vi "(FPGA)_PIDXYZ_laserPID)_COMtemp2.vi"() -> ()   [LabVIEW 2018]
doc: "This VI will read single point values from 4 channels of a R Series board at a specified rate."
uses:
  <vilib>/rvi/Emulation/niFpgaGetClockAttributes.vi
  <vilib>/rvi/Emulation/niFpgaSctlEmulationGetInTimedLoop.vi
  <vilib>/rvi/Emulation/niFpgaEmulationReportErrorSimple.vi
  <vilib>/rvi/eio/common/nirviEmuTemplateMethod_errors.vi
  <vilib>/rvi/Emulation/niFpgaProcessEmulError.vi
  <vilib>/rvi/Emulation/niFpgaCriticalErrorInLSC.vi
  <vilib>/rvi/Memory/Memory_Emulation/nirvimemoryFastEmulation.vi
  <vilib>/rvi/Memory/Memory_Emulation/nirvimemoryEmulation.vi
  <vilib>/rvi/Emulation/niFpgaEmulationIsFPGAContextNoSignature.vi
  <vilib>/rvi/DataTransferAndStorage/Container/Common/niFpgaContainerGetUniqueNameForEmu.vi
  <vilib>/rvi/errors/nirviReportUnexpectedCaseInternalError (U32).vi
  <vilib>/rvi/Memory/Memory_Emulation/niFpgaMemoryEmulationCacheClearOnFirstRun.vi
  <vilib>/rvi/Memory/Memory_Emulation/nirvimemoryEmulationManagerCache_MakeExclusive.vi
  <vilib>/rvi/Memory/Memory_Emulation/niFpgaMemoryEmulationValidateCache.vi
  <vilib>/rvi/Memory/Memory_Emulation/nirvimemoryEmulationManagerCache_InsertValue.vi
  <vilib>/Utility/error.llb/Clear Errors.vi
  <vilib>/rvi/Memory/Memory_Emulation/nirvimemoryEmulationManagerCache_ReleaseExclusive.vi
  <vilib>/rvi/Memory/Memory_Emulation/nirvimemoryEmulationManagerCache_GetValue.vi
  <vilib>/rvi/Memory/Memory_Emulation/nirvimemoryEmulationManagerCache_SetValue.vi
  <vilib>/rvi/Emulation/niFpgaSctlEmulationResourceMgr.vi
  <vilib>/eio/EIONode/EIONode.xnode
  <vilib>/rvi/DataTransferAndStorage/Container/XNode/niFpgaContainer.xnode
  <vilib>/rvi/FXPMathLib/FxpInterpret/XNode/nifxpmath_Interpret.xnode
panel:
  in  "Amplitude AO7":fxp<+/-,64,32>
  in  "Amplitude AO6":fxp<+/-,64,32>
  in  "Amplitude AO5":fxp<+/-,64,32>
  in  "Amplitude AO4":fxp<+/-,64,32>
  in  "phase offset AO7":fxp<+,32,0>
  in  "reset AO7":bool
  in  "frequency AO7":fxp<+,32,0>=0.0002500000409781933
  in  "phase offset AO6":fxp<+,32,0>
  in  "reset AO6":bool
  in  "frequency AO6":fxp<+,32,0>=0.0002500000409781933
  in  "phase offset AO5":fxp<+,32,0>
  in  "reset AO5":bool
  in  "frequency AO5":fxp<+,32,0>=0.0002500000409781933
  in  "phase offset AO4":fxp<+,32,0>
  in  "reset AO4":bool
  in  "frequency AO4":fxp<+,32,0>=0.0002500000409781933
  in  "stop":bool
  in  "Notch coeff y 2":i32[](array[numeric])=[-1060332860, 1067037342, -2129863576]
  in  "Notch coeff y 1":i32[](array[numeric])=[-1060332860, 1067037342, -2129863576]
  in  "Notch coeff x":i32[](array[numeric])=[-1060332860, 1067037342, -2129863576]
  out "accum out z2":fxp<+/-,37,37>
  out "accurm reset z2":bool
  out "accum out z1":fxp<+/-,37,37>
  out "accum reset z1":bool
  in  "Reset x accum":bool
  in  "Reset y accum":bool
  in  "Reset z accum":bool
  out "master y":bool
  out "master x":bool
  in  "No_integral_gain":bool=TRUE
  in  "Y_emergency_threshould":i16
  in  "X_emergency_threshould":i16
  in  "Big Number":sgl
  in  "Amplitude_sine_EOM":sgl
  in  "eom sine frequency (periods/tick)":fxp<+,32,0>=0.0002500000409781933
  in  "pz?":bool
  out "pg Z mod":fxp<+/-,24,12>
  in  "pg Z":fxp<+/-,24,12>
  in  "amplitude":i16=8192
  in  "offset":i16=8192
  out "Trigger for COM out":i16 caption="square wave out"
  out "dgz mod":fxp<+/-,24,12>
  in  "activate COMz":bool
  in  "dg Z":fxp<+/-,24,12>
  in  "activate COMy":bool
  out "dgy mod":fxp<+/-,24,12>
  in  "dg Y":fxp<+/-,24,12>
  out "dgx mod":fxp<+/-,24,12>
  in  "activate COMx":bool
  in  "dg X":fxp<+/-,24,12>
  in  "duty cycle (periods)":fxp<+,32,0>=0.5
  in  "frequency (periods/tick)":fxp<+,32,0>=0.00390625
  in  "final filter coeff X before":i32[](array[numeric])=[-955995012, 2025731616, 1001305, -1023351008, 2092954700, 1034533]
  in  "final filter coeff X":i32[](array[numeric])=[-955995012, 2025731616, 1001305, -1023351008, 2092954700, 1034533]
  in  "final filter coeff Y before":i32[](array[numeric])=[-955995012, 2025731616, 1001305, -1023351008, 2092954700, 1034533]
  in  "final filter coeff Y":i32[](array[numeric])=[-955995012, 2025731616, 1001305, -1023351008, 2092954700, 1034533]
  in  "final filter coeff Z":i32[](array[numeric])=[-955995012, 2025731616, 1001305, -1023351008, 2092954700, 1034533]
  in  "final filter coeff Z before":i32[](array[numeric])=[-955995012, 2025731616, 1001305, -1023351008, 2092954700, 1034533]
  in  "LP Coeff Z before":i32[](array[numeric])=[1008310688, 32715568]
  in  "LP Coeff Z":i32[](array[numeric])=[1008310688, 32715568]
  in  "LP Coeff X":i32[](array[numeric])=[1008310688, 32715568]
  in  "LP Coeff X before":i32[](array[numeric])=[1008310688, 32715568]
  in  "LP Coeff Y before":i32[](array[numeric])=[1008310688, 32715568]
  in  "LP Coeff Y":i32[](array[numeric])=[1008310688, 32715568]
  in  "Upper lim Z before":fxp<+/-,16,16>
  in  "Lower lim Z before":fxp<+/-,16,16>
  in  "Upper lim Y before":fxp<+/-,16,16>
  in  "Lower lim Y before":fxp<+/-,16,16>
  in  "Upper lim X before":fxp<+/-,16,16>
  in  "Lower lim X before":fxp<+/-,16,16>
  in  "HP coeff band X before":i32[](array[numeric])=[-850883994, 1909449570, 958518847, -975456236, 2033039520, 1020559395]
  in  "LP Coeff band X before":i32[](array[numeric])=[-955995012, 2025731616, 1001305, -1023351008, 2092954700, 1034533]
  in  "LP Coeff band X":i32[](array[numeric])=[-955995012, 2025731616, 1001305, -1023351008, 2092954700, 1034533]
  in  "HP Coeff band X":i32[](array[numeric])=[-850883994, 1909449570, 958518847, -975456236, 2033039520, 1020559395]
  in  "dg band X before":fxp<+/-,24,12>
  in  "dg band X":fxp<+/-,24,12>
  in  "HP Coeff X before":i32[](array[numeric])=[946630756, 1010186290]
  in  "HP Coeff X":i32[](array[numeric])=[946630756, 1010186290]
  in  "Use X PID before":bool
  out "AI X before chamber plot":i16
  in  "X before Setpoint":i16
  out "tot_fb X plot":i16
  out "fb X before chamber plot":i16
  in  "DC offset X":i16
  in  "pg X before":fxp<+/-,24,12>
  in  "ig X before":fxp<+/-,24,-4>
  in  "dg X before":fxp<+/-,24,12>
  out "fb X plot":i16
  in  "ig X":fxp<+/-,24,-4>
  in  "Lower lim X":fxp<+/-,16,16>
  in  "Upper lim X":fxp<+/-,16,16>
  in  "pg X":fxp<+/-,24,12>
  out "AI X plot":i16
  in  "X Setpoint":i16
  in  "HP coeff band Y before":i32[](array[numeric])=[-850883994, 1909449570, 958518847, -975456236, 2033039520, 1020559395]
  in  "LP Coeff band Y before":i32[](array[numeric])=[-955995012, 2025731616, 1001305, -1023351008, 2092954700, 1034533]
  in  "LP Coeff band Y":i32[](array[numeric])=[-955995012, 2025731616, 1001305, -1023351008, 2092954700, 1034533]
  in  "HP Coeff band Y":i32[](array[numeric])=[-850883994, 1909449570, 958518847, -975456236, 2033039520, 1020559395]
  in  "dg band Y before":fxp<+/-,24,12>
  in  "dg band Y":fxp<+/-,24,12>
  in  "HP Coeff Y before":i32[](array[numeric])=[946630756, 1010186290]
  in  "HP Coeff Y":i32[](array[numeric])=[946630756, 1010186290]
  in  "Use Y PID before":bool
  out "AI Y before chamber plot":i16
  in  "Y before Setpoint":i16
  out "tot_fb Y plot":i16
  out "fb Y before chamber plot":i16
  in  "DC offset Y":i16
  in  "pg Y before":fxp<+/-,24,12>
  in  "ig Y before":fxp<+/-,24,-4>
  in  "dg Y before":fxp<+/-,24,12>
  out "fb Y plot":i16
  in  "ig Y":fxp<+/-,24,-4>
  in  "Lower lim Y":fxp<+/-,16,16>
  in  "Upper lim Y":fxp<+/-,16,16>
  in  "pg Y":fxp<+/-,24,12>
  out "AI Y plot":i16
  in  "Y Setpoint":i16
  in  "EOM_offset":i16
  in  "EOM_seed":u32=4294967295 caption="seed"
  in  "EOM reset":bool caption="reset"
  in  "EOM_threshold":i16
  in  "EOM_amplitude":i16
  in  "HP coeff band Z before":i32[](array[numeric])=[-850883994, 1909449570, 958518847, -975456236, 2033039520, 1020559395]
  in  "LP Coeff band Z before":i32[](array[numeric])=[-955995012, 2025731616, 1001305, -1023351008, 2092954700, 1034533]
  in  "LP Coeff band Z":i32[](array[numeric])=[-955995012, 2025731616, 1001305, -1023351008, 2092954700, 1034533]
  in  "HP Coeff band Z":i32[](array[numeric])=[-850883994, 1909449570, 958518847, -975456236, 2033039520, 1020559395]
  in  "dg band Z before":fxp<+/-,24,12>
  in  "dg band Z":fxp<+/-,24,12>
  in  "data_buffer3":i16
  in  "Arb gain (ch2)":fxp<+/-,24,12>=0.5 caption="RMS"
  in  "HP Coeff Z before":i32[](array[numeric])=[946630756, 1010186290]
  in  "HP Coeff Z":i32[](array[numeric])=[946630756, 1010186290]
  in  "Use Z PID before":bool
  out "AI Z before chamber plot":i16
  in  "Z before Setpoint":i16
  out "tot_fb Z plot":i16
  out "fb Z before chamber plot":i16
  in  "DC offset Z":i16
  in  "pg Z before":fxp<+/-,24,12>
  in  "ig Z before":fxp<+/-,24,-4>
  in  "dg Z before":fxp<+/-,24,12>
  out "fb Z plot":i16
  in  "ig Z":fxp<+/-,24,-4>
  out "written_address":u32
  in  "ready_to_write":bool
  in  "Arb steps per cycle":u16
  in  "data_buffer2":i16
  in  "data_buffer_1":i16
  in  "write_address":u16
  in  "Arb gain (ch1)":fxp<+/-,24,12>=0.5 caption="RMS"
  in  "Arb gain (ch0)":fxp<+/-,24,12>=0.5 caption="RMS"
  in  "Lower lim Z":fxp<+/-,16,16>
  in  "Upper lim Z":fxp<+/-,16,16>
  out "AI Z plot":i16
  in  "Z Setpoint":i16
  in  "Count(uSec)":u32
  out "FPGA Error Out":errorcluster
  in  "Stop":bool
  # "test"
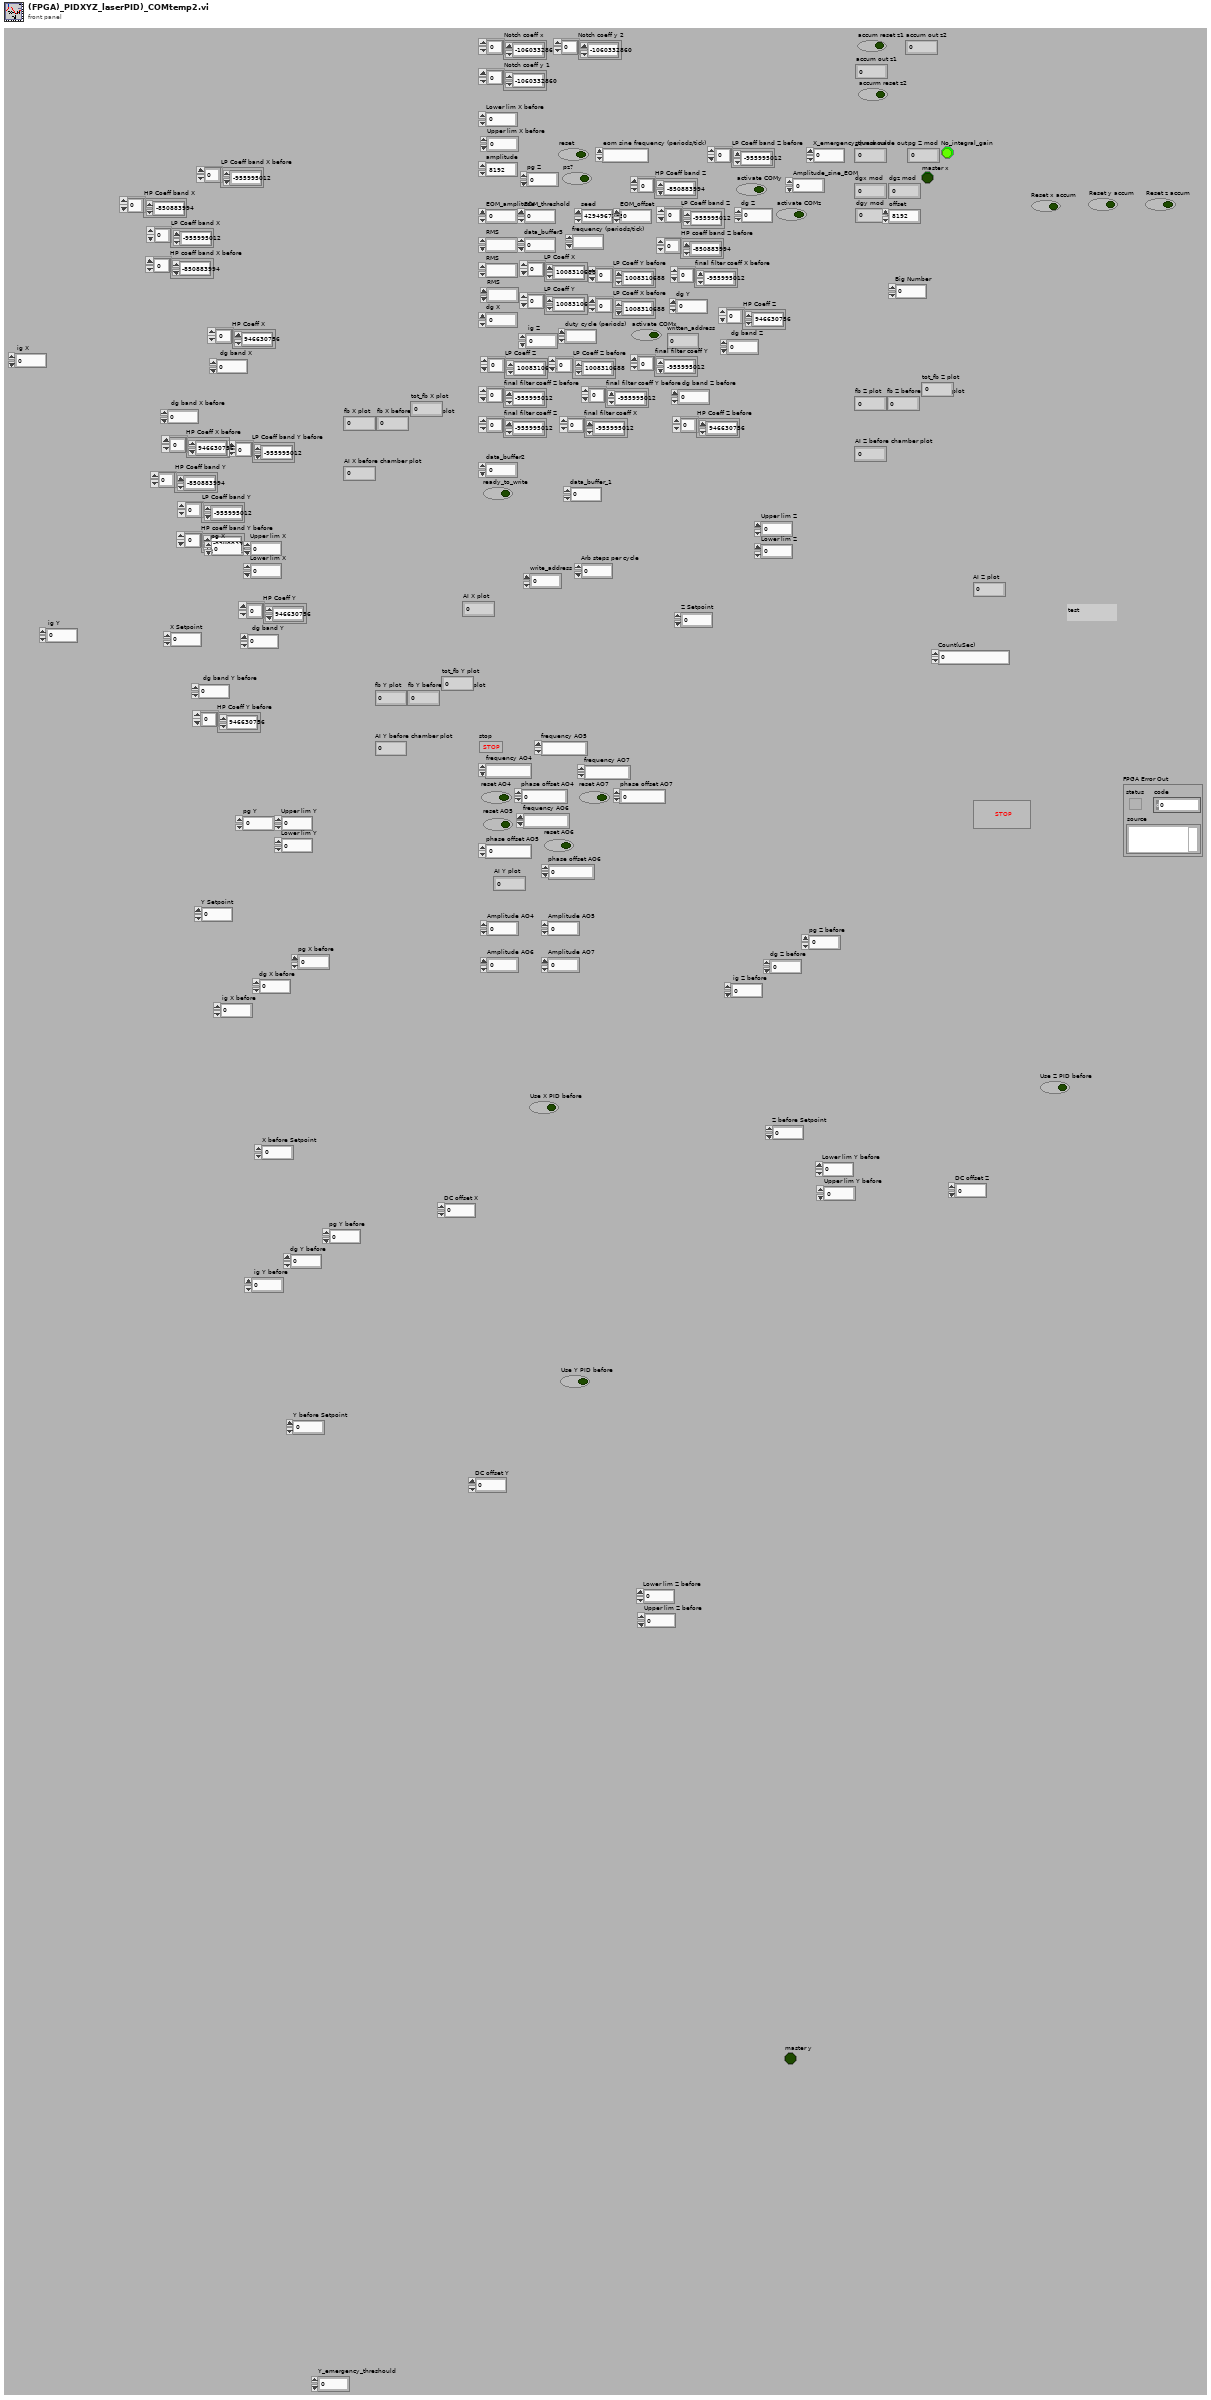
[diagram p1: front panel]
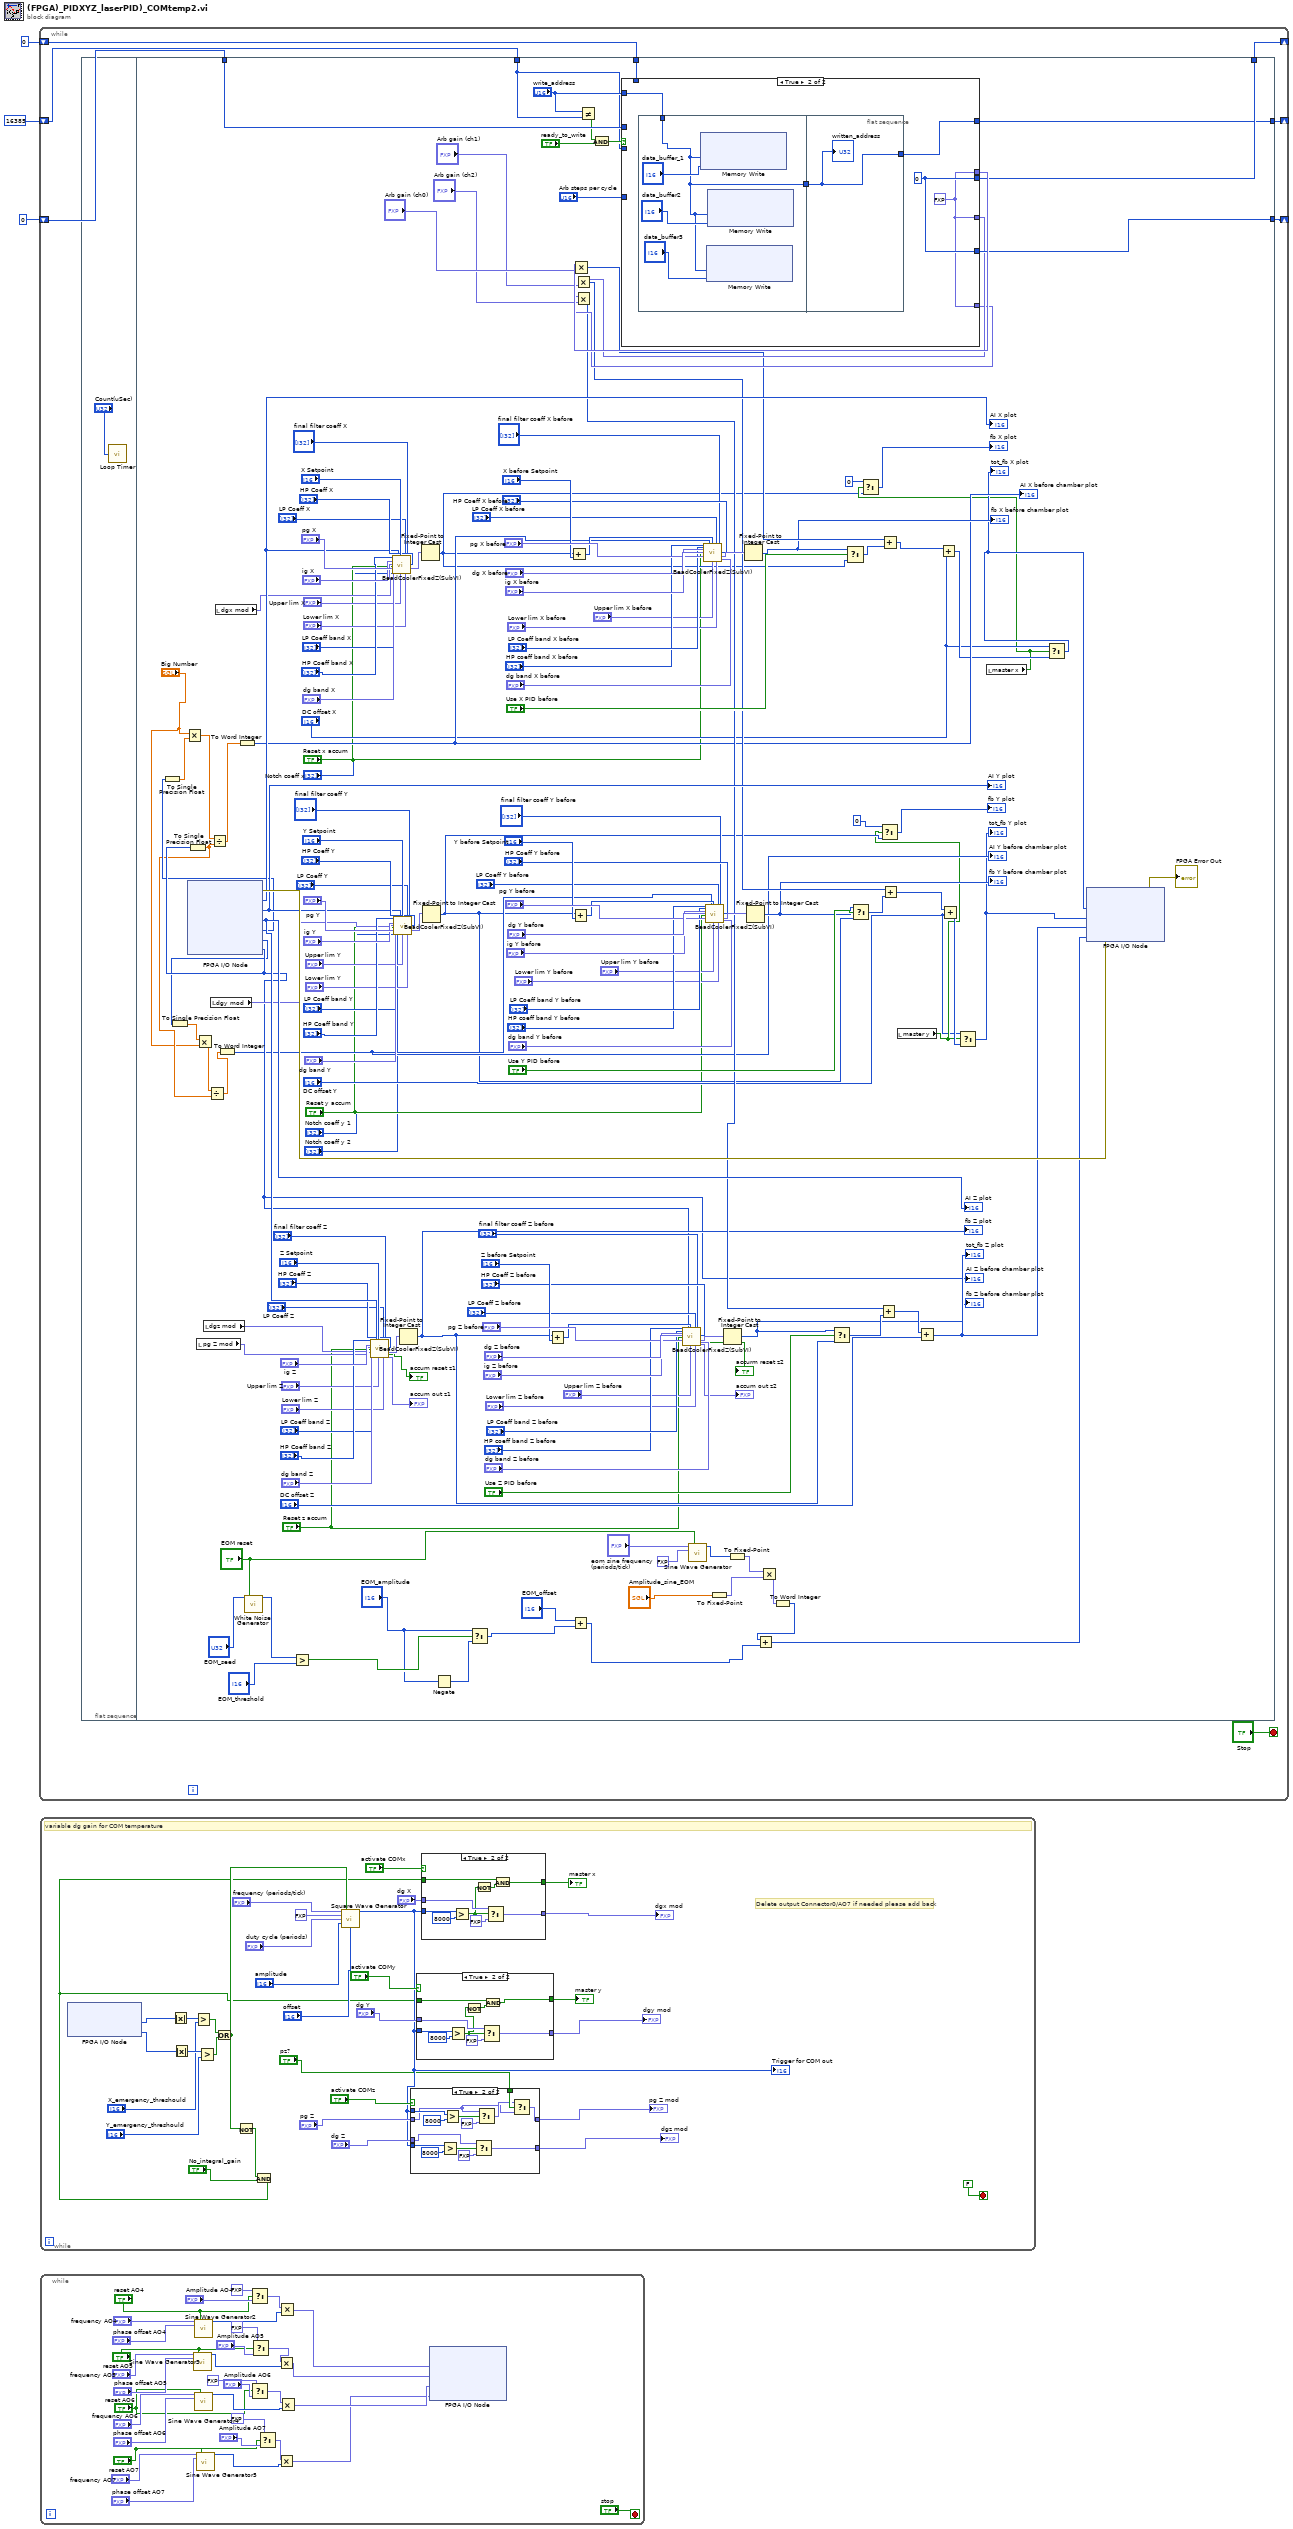
[diagram p0: block diagram]
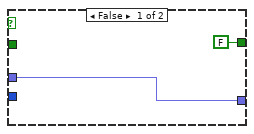
[diagram p3: hidden frame]
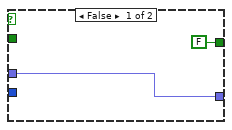
[diagram p4: hidden frame]
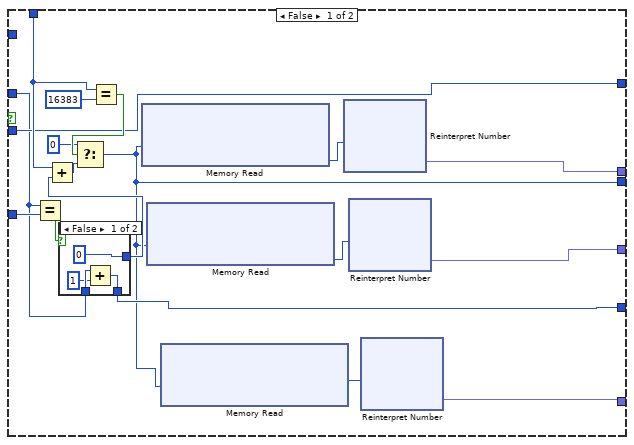
[diagram p5: hidden frame]
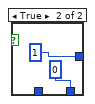
[diagram p6: hidden frame]
diagram:
  n1 = while {
    shift-right: [w9] -> _
    shift-left: u16 0 ("t") -> [w8]
    shift-right: [w7] -> _
    shift-left: u16 0 ("t") -> [w4]
    shift-right: [w6] -> _
    shift-left: u32 16385 ("write_address") -> [w5]
    stop <- "Stop" stop-if-true
    n2 = flat-sequence {
      tunnel: [w183] -> w9
      tunnel: w8 -> [w182]
      tunnel: [w180] -> w7
      tunnel: w4 -> [w179]
      tunnel: [w178] -> w6
      tunnel: w5 -> [w171]
      frame #0 {
        n3 = call "Loop Timer"("Count(uSec)"="Count(uSec)") -> ()  [unwired: 1 out]
      }
      frame #1 {
        n4 = xnode "FPGA I/O Node"() -> ("error out"=w188:errorcluster, "Connector0/AI0"=w95:i16, "Connector0/AI1"=w117:i16, "Connector0/AI2"=w169:i16, "Connector0/AI3"=w43:i16, "Connector0/AI4"=w42:i16, "Connector0/AI5"=w47:i16)  [unwired: 7 in, 6 out]
        "AI Z plot" <- w169
        "AI Z before chamber plot" <- w47
        "AI Y plot" <- w117
        "AI X plot" <- w95
        n5 = To Single Precision Float(number=w43) -> (single precision float=w46:sgl)
        n6 = To Single Precision Float(number=w42) -> (single precision float=w41:sgl)
        n7 = Multiply(x="Big Number", y=w46) -> (x*y=w45:sgl)
        n8 = To Single Precision Float(number=w47) -> (single precision float=w39:sgl)
        n9 = Multiply(x=w41, y="Big Number") -> (x*y=w40:sgl)
        n10 = local read "pg Z mod"() -> (w60:fxp<+/-,24,12>)
        n11 = local read "dgz mod"() -> (w61:fxp<+/-,24,12>)
        n12 = Divide(x=w40, y=w39) -> (x/y=w38:sgl)
        n13 = Divide(x=w45, y=w39) -> (x/y=w44:sgl)
        n14 = local read "dgy mod"() -> (w62:fxp<+/-,24,12>)
        n15 = local read "dgx mod"() -> (w63:fxp<+/-,24,12>)
        n16 = To Word Integer(number=w38) -> (16bit integer=w37:i16)
        "AI Y before chamber plot" <- w37
        n17 = To Word Integer(number=w44) -> (16bit integer=w48:i16)
        "AI X before chamber plot" <- w48
        n18 = call "White Noise Generator"("seed"="EOM_seed", "reset"="EOM reset") -> ("white noise out"=w148:i16)  [unwired: 13 in]
        n19 = Greater?(x=w148, y="EOM_threshold") -> (0:w146:bool)
        n20 = call "BeadCoolerFixedZ(SubVI).vi"("hp coeff band"="HP Coeff band Z", "lp coeff band"="LP Coeff band Z", "ig"="ig Z", "dg"=w61, "load (F)"="Reset z accum", "pg"=w60, "dg band"="dg band Z", "AI0"=w169, "Dc Pos"="Z Setpoint", "Upper lim"="Upper lim Z", "lp coeff"="LP Coeff Z", "Lower lim"="Lower lim Z", "final filter coeff"="final filter coeff Z", "hp coeff"="HP Coeff Z") -> ("Output"=w158:fxp<+/-,16,16>, "accurm reset"=→"accum reset z1":bool, "accum out"=→"accum out z1":fxp<+/-,37,37>)  [unwired: 11 in]
        n21 = call "BeadCoolerFixedZ(SubVI).vi"("hp coeff band"="HP Coeff band X", "lp coeff band"="LP Coeff band X", "ig"="ig X", "dg"=w63, "load (F)"="Reset x accum", "pg"="pg X", "dg band"="dg band X", "Notch coeff 1"="Notch coeff x", "AI0"=w95, "Dc Pos"="X Setpoint", "Upper lim"="Upper lim X", "lp coeff"="LP Coeff X", "Lower lim"="Lower lim X", "final filter coeff"="final filter coeff X", "hp coeff"="HP Coeff X") -> ("Output"=w105:fxp<+/-,16,16>)  [unwired: 10 in, 2 out]
        n22 = call "BeadCoolerFixedZ(SubVI).vi"("hp coeff band"="HP Coeff band Y", "lp coeff band"="LP Coeff band Y", "ig"="ig Y", "dg"=w62, "load (F)"="Reset y accum", "pg"="pg Y", "dg band"="dg band Y", "Notch coeff 1"="Notch coeff y 1", "Notch coeff 2"="Notch coeff y 2", "AI0"=w117, "Dc Pos"="Y Setpoint", "Upper lim"="Upper lim Y", "lp coeff"="LP Coeff Y", "Lower lim"="Lower lim Y", "final filter coeff"="final filter coeff Y", "hp coeff"="HP Coeff Y") -> ("Output"=w127:fxp<+/-,16,16>)  [unwired: 9 in, 2 out]
        n23 = Fixed-Point to Integer Cast(1:w158) -> (0:w73:i16)
        "fb Z plot" <- w73
        n24 = Fixed-Point to Integer Cast(1:w105) -> (0:w23:i16)
        n25 = Fixed-Point to Integer Cast(1:w127) -> (0:w31:i16)
        n26 = Negate(x="EOM_amplitude") -> (-x=w144:i16)
        n27 = Select(t="EOM_amplitude", s=w146, f=w144) -> (s? t:f=w142:i16)
        n28 = Add(x=w73, y="Z before Setpoint") -> (x+y=w157:i16)
        n29 = Add(x=w23, y="X before Setpoint") -> (x+y=w104:i16)
        n30 = Add(x=w31, y="Y before Setpoint") -> (x+y=w126:i16)
        n31 = Add(x="EOM_offset", y=w142) -> (x+y=w51:i16)
        n32 = Not Equal?(x="write_address", y=w171) -> (x != y?=w175:bool)
        n33 = And(x=w175, y="ready_to_write") -> (x .and. y?=w176:bool)
        n34 = case shown="True" w176 {
          tunnel: [w205 w213] -> w185
          tunnel: [w190 w217] -> w183
          tunnel: w182 -> [w198 _]
          tunnel: [w199 w213] -> w173
          tunnel: "Arb steps per cycle" -> [w197 _]
          tunnel: [w192 w217] -> w180
          tunnel: w179 -> [w193 _]
          tunnel: [w196 w215] -> w178
          tunnel: w171 -> [w196 _]
          tunnel: "write_address" -> [_ w214]
          tunnel: [w189 w213] -> w155
          frame False {
            n35 = Equal?(x=w193, y=w197) -> (x = y?=w195:bool)
            n36 = case shown="False" w195 {
              tunnel: [u16 0 ("y") u16 1 ("y")] -> w194
              tunnel: w193 -> [w209 _]
              tunnel: [w207 u16 0] -> w192
              frame False {
                n37 = Add(x=w209, y=u16 1) -> (x+y=w207:u16)
              }
              frame True {
              }
            }
            n38 = Add(x=w198, y=w194) -> (x+y=w201:u16)
            n39 = Equal?(x=w198, y=u16 16383) -> (x = y?=w203:bool)
            n40 = Select(t=u16 0, s=w203, f=w201) -> (s? t:f=w190:u16)
            n41 = xnode ("Memory Read")("Address"=w190) -> ("Data"=w206:i16)  [unwired: 1 in, 1 out]
            n42 = xnode ("Memory Read")("Address"=w190) -> ("Data"=w200:i16)  [unwired: 1 in, 1 out]
            n43 = xnode ("Memory Read")("Address"=w190) -> ("Data"=w191:i16)  [unwired: 1 in, 1 out]
            n44 = xnode "Reinterpret Number"("x"=w206) -> ("y"=w205:fxp<+/-,16,16>)
            n45 = xnode "Reinterpret Number"("x"=w200) -> ("y"=w199:fxp<+/-,16,16>)
            n46 = xnode "Reinterpret Number"("x"=w191) -> ("y"=w189:fxp<+/-,16,16>)
          }
          frame True {
            w217 = u16 0
            w213 = fxp<+/-,16,16> 0.0 ("y")
            n47 = flat-sequence {
              tunnel: [w219] -> w216
              tunnel: w214 -> [w219]
              tunnel: w216 -> [w222]
              tunnel: [w222] -> w215
              frame #0 {
                n48 = xnode ("Memory Write")("Address"=w219, "Data"="data_buffer_1") -> ()  [unwired: 1 in, 1 out]
                n49 = xnode ("Memory Write")("Address"=w219, "Data"="data_buffer3") -> ()  [unwired: 1 in, 1 out]
                n50 = xnode ("Memory Write")("Address"=w219, "Data"="data_buffer2") -> ()  [unwired: 1 in, 1 out]
              }
              frame #1 {
                "written_address" <- w222
              }
            }
          }
        }
        n51 = Multiply(x=w185, y="Arb gain (ch0)") -> (x*y=w76:i16)
        n52 = Multiply(x=w173, y="Arb gain (ch1)") -> (x*y=w75:i16)
        n53 = Multiply(x=w155, y="Arb gain (ch2)") -> (x*y=w74:i16)
        n54 = call "BeadCoolerFixedZ(SubVI).vi"("hp coeff band"="HP coeff band Z before", "lp coeff band"="LP Coeff band Z before", "ig"="ig Z before", "dg"="dg Z before", "load (F)"="Reset z accum", "pg"="pg Z before", "dg band"="dg band Z before", "AI0"=w47, "Dc Pos"=w157, "Upper lim"="Upper lim Z before", "lp coeff"="LP Coeff Z before", "Lower lim"="Lower lim Z before", "final filter coeff"="final filter coeff Z before", "hp coeff"="HP Coeff Z before") -> ("Output"=w165:fxp<+/-,16,16>, "accurm reset"=→"accurm reset z2":bool, "accum out"=→"accum out z2":fxp<+/-,37,37>)  [unwired: 11 in]
        n55 = call "Sine Wave Generator"("frequency (periods/tick)"="eom sine frequency (periods/tick)", "reset"="EOM reset", "phase offset (periods)"=fxp<+,32,0> 0.0) -> ("sine out"=w57:i16)  [unwired: 12 in]
        n56 = call "BeadCoolerFixedZ(SubVI).vi"("hp coeff band"="HP coeff band X before", "lp coeff band"="LP Coeff band X before", "ig"="ig X before", "dg"="dg X before", "load (F)"="Reset x accum", "pg"="pg X before", "dg band"="dg band X before", "AI0"=w48, "Dc Pos"=w104, "Upper lim"="Upper lim X before", "lp coeff"="LP Coeff X before", "Lower lim"="Lower lim X before", "final filter coeff"="final filter coeff X before", "hp coeff"="HP Coeff X before") -> ("Output"=w110:fxp<+/-,16,16>)  [unwired: 11 in, 2 out]
        n57 = call "BeadCoolerFixedZ(SubVI).vi"("hp coeff band"="HP coeff band Y before", "lp coeff band"="LP Coeff band Y before", "ig"="ig Y before", "dg"="dg Y before", "load (F)"="Reset y accum", "pg"="pg Y before", "dg band"="dg band Y before", "AI0"=w37, "Dc Pos"=w126, "Upper lim"="Upper lim Y before", "lp coeff"="LP Coeff Y before", "Lower lim"="Lower lim Y before", "final filter coeff"="final filter coeff Y before", "hp coeff"="HP Coeff Y before") -> ("Output"=w132:fxp<+/-,16,16>)  [unwired: 11 in, 2 out]
        n58 = To Fixed-Point(number="Amplitude_sine_EOM") -> (fixed-point=w55:fxp<+/-,32,16>)  [unwired: 1 in]
        n59 = Fixed-Point to Integer Cast(1:w165) -> (0:w64:i16)
        "fb Z before chamber plot" <- w64
        n60 = To Fixed-Point(number=w57) -> (fixed-point=w56:fxp<+/-,16,16>)  [unwired: 1 in]
        n61 = Fixed-Point to Integer Cast(1:w110) -> (0:w70:i16)
        "fb X before chamber plot" <- w70
        n62 = Fixed-Point to Integer Cast(1:w132) -> (0:w67:i16)
        "fb Y before chamber plot" <- w67
        n63 = Multiply(x=w56, y=w55) -> (x*y=w54:fxp<+/-,48,32>)
        n64 = To Word Integer(number=w54) -> (16bit integer=w52:i16)
        n65 = Add(x=w52, y=w51) -> (x+y=w50:i16)
        n66 = Select(t=w64, s="Use Z PID before", f=w73) -> (s? t:f=w66:i16)
        n67 = Select(t=w70, s="Use X PID before", f=w23) -> (s? t:f=w72:i16)
        n68 = Select(t=w67, s="Use Y PID before", f=w31) -> (s? t:f=w69:i16)
        n69 = Add(x=w74, y=w66) -> (x+y=w65:i16)
        n70 = Add(x=w76, y=w72) -> (x+y=w71:i16)
        n71 = Add(x=w75, y=w69) -> (x+y=w68:i16)
        n72 = local read "master y"() -> (w30:bool)
        n73 = Select(t=i16 0, s=w30, f=w31) -> (s? t:f=→"fb Y plot":i16)
        n74 = Add(x=w65, y="DC offset Z") -> (x+y=w161:i16)
        "tot_fb Z plot" <- w161
        n75 = Add(x=w71, y="DC offset X") -> (x+y=w28:i16)
        n76 = Add(x=w68, y="DC offset Y") -> (x+y=w35:i16)
        n77 = Select(t="DC offset Y", s=w30, f=w35) -> (s? t:f=w34:i16)
        "tot_fb Y plot" <- w34
        n78 = local read "master x"() -> (w25:bool)
        n79 = Select(t=i16 0, s=w25, f=w23) -> (s? t:f=→"fb X plot":i16)
        n80 = Select(t="DC offset X", s=w25, f=w28) -> (s? t:f=w27:i16)
        "tot_fb X plot" <- w27
        n81 = xnode "FPGA I/O Node"("error in"=w188, "Connector0/AO0"=w27, "Connector0/AO1"=w34, "Connector0/AO2"=w161, "Connector0/AO3"=w50) -> ("error out"=→"FPGA Error Out":errorcluster)  [unwired: 4 in, 4 out]
      }
    }
  }
  n82 = while {
    stop <- FALSE stop-if-true
    # "Delete output Connector0/AO7 if needed please add back"
    # "variable dg gain for COM temperature"
    n83 = xnode "FPGA I/O Node"() -> ("Connector0/AI0"=w236:i16, "Connector0/AI1"=w235:i16)  [unwired: 3 in, 3 out]
    n84 = Absolute Value(x=w236) -> (abs(x)=w234:i16)
    n85 = Absolute Value(x=w235) -> (abs(x)=w233:i16)
    n86 = Greater?(x=w234, y="X_emergency_threshould") -> (0:w230:bool)
    n87 = Greater?(x=w233, y="Y_emergency_threshould") -> (0:w229:bool)
    n88 = Or(x=w230, y=w229) -> (x .or. y?=w228:bool)
    n89 = Not(x=w228) -> (.not. x?=w227:bool)
    n90 = And(x=w227, y="No_integral_gain") -> (x .and. y?=w225:bool)
    n91 = call "Square Wave Generator"("frequency (periods/tick)"="frequency (periods/tick)", "reset"=w228, "phase offset (periods)"=fxp<+,32,0> 0.0, "duty cycle (periods)"="duty cycle (periods)", "amplitude"="amplitude", "offset"="offset") -> ("square wave out"=w238:i16)  [unwired: 9 in]
    "Trigger for COM out" <- w238
    n92 = case shown="True" "activate COMz" {
      tunnel: [w257 w268] -> w241
      tunnel: w238 -> [_ w271]
      tunnel: "dg Z" -> [w257 w266]
      tunnel: "pg Z" -> [w256 w258]
      tunnel: [w256 w259] -> w239
      tunnel: w238 -> [_ w262]
      tunnel: "pz?" -> [_ w261]
      frame False {
      }
      frame True {
        n93 = Greater?(x=w271, y=i16 8000) -> (0:w269:bool)
        n94 = Greater?(x=w262, y=i16 8000) -> (0:w264:bool)
        n95 = Select(t=w266, s=w269, f=fxp<+/-,24,12> 0.0 ("y")) -> (s? t:f=w268:fxp<+/-,24,12>)
        n96 = Select(t=w258, s=w264, f=fxp<+/-,24,12> 0.0 ("y")) -> (s? t:f=w260:fxp<+/-,24,12>)
        n97 = Select(t=w260, s=w261, f=w258) -> (s? t:f=w259:fxp<+/-,24,12>)
      }
    }
    "dgz mod" <- w241
    "pg Z mod" <- w239
    n98 = case shown="True" "activate COMy" {
      tunnel: "dg Y" -> [w273 w279]
      tunnel: [w273 w280] -> w245
      tunnel: w238 -> [_ w282]
      tunnel: w225 -> [_ w276]
      tunnel: [FALSE w274] -> w223
      frame False {
      }
      frame True {
        n99 = Greater?(x=w282, y=i16 8000) -> (0:w275:bool)
        n100 = Not(x=w275) -> (.not. x?=w277:bool)
        n101 = Select(t=w279, s=w275, f=fxp<+/-,24,12> 0.0 ("y")) -> (s? t:f=w280:fxp<+/-,24,12>)
        n102 = And(x=w276, y=w277) -> (x .and. y?=w274:bool)
      }
    }
    "dgy mod" <- w245
    "master y" <- w223
    n103 = case shown="True" "activate COMx" {
      tunnel: "dg X" -> [w284 w290]
      tunnel: [w284 w291] -> w247
      tunnel: w238 -> [_ w293]
      tunnel: w225 -> [_ w286]
      tunnel: [FALSE w285] -> w224
      frame False {
      }
      frame True {
        n104 = Greater?(x=w293, y=i16 8000) -> (0:w288:bool)
        n105 = Not(x=w288) -> (.not. x?=w287:bool)
        n106 = Select(t=w290, s=w288, f=fxp<+/-,24,12> 0.0 ("y")) -> (s? t:f=w291:fxp<+/-,24,12>)
        n107 = And(x=w286, y=w287) -> (x .and. y?=w285:bool)
      }
    }
    "dgx mod" <- w247
    "master x" <- w224
  }
  n108 = while {
    stop <- "stop" stop-if-true
    n109 = call "Sine Wave Generator3"("frequency (periods/tick)"="frequency AO5", "reset"="reset AO5", "phase offset (periods)"="phase offset AO5") -> ("sine out"=w315:i16)  [unwired: 12 in]
    n110 = call "Sine Wave Generator2"("frequency (periods/tick)"="frequency AO4", "reset"="reset AO4", "phase offset (periods)"="phase offset AO4") -> ("sine out"=w317:i16)  [unwired: 12 in]
    n111 = call "Sine Wave Generator4"("frequency (periods/tick)"="frequency AO6", "reset"="reset AO6", "phase offset (periods)"="phase offset AO6") -> ("sine out"=w313:i16)  [unwired: 12 in]
    n112 = call "Sine Wave Generator5"("frequency (periods/tick)"="frequency AO7", "reset"="reset AO7", "phase offset (periods)"="phase offset AO7") -> ("sine out"=w311:i16)  [unwired: 12 in]
    n113 = Select(t=fxp<+/-,64,32> 0.0, s="reset AO4", f="Amplitude AO4") -> (s? t:f=w294:fxp<+/-,64,32>)
    n114 = Select(t=fxp<+/-,64,32> 0.0, s="reset AO6", f="Amplitude AO6") -> (s? t:f=w299:fxp<+/-,64,32>)
    n115 = Select(t=fxp<+/-,64,32> 0.0, s="reset AO5", f="Amplitude AO5") -> (s? t:f=w303:fxp<+/-,64,32>)
    n116 = Select(t=fxp<+/-,64,32> 0.0, s="reset AO7", f="Amplitude AO7") -> (s? t:f=w295:fxp<+/-,64,32>)
    n117 = Multiply(x=w303, y=w315) -> (x*y=w314:fxp<+/-,64,48>)
    n118 = Multiply(x=w295, y=w311) -> (x*y=w310:fxp<+/-,64,48>)
    n119 = Multiply(x=w294, y=w317) -> (x*y=w316:fxp<+/-,64,48>)
    n120 = Multiply(x=w299, y=w313) -> (x*y=w312:fxp<+/-,64,48>)
    n121 = xnode "FPGA I/O Node"("Connector0/AO4"=w316, "Connector0/AO5"=w314, "Connector0/AO6"=w312, "Connector0/AO7"=w310) -> ()  [unwired: 5 in, 5 out]
  }
